vi "power_to_voltage.vi"(1 "Power (%)":dbl) -> (0 "Voltage":dbl[](array[numeric]))   [LabVIEW 2020]
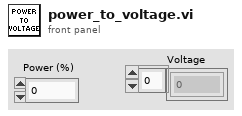
[diagram p1: front panel]
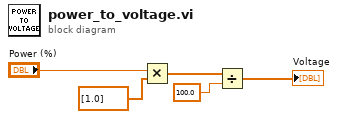
[diagram p0: block diagram]
diagram:
  n1 = Multiply(x="Power (%)", y=dbl[] [1.0] ("data")) -> (x*y=w3:dbl[])
  n2 = Divide(x=w3, y=100.0) -> (x/y=→"Voltage":dbl[])
